vi "Write Voltage Setting.vi"(0 "VISA resource name":refnum<visa-resource-name>, 1 "Enable Voltage Inversion (T: Enabled)":bool=TRUE, 7 "Voltage Setting (100.00)":dbl=100.0 format="%.2f", 11 "error in (no error)":errorcluster) -> (4 "VISA resource name out":refnum<visa-resource-name>, 15 "error out":errorcluster)   [LabVIEW 2011, in "Stanford Research PS300 Series.lvlib"]
doc: "This VI sets the output value and causes the instrument to output voltage."
uses:
  <instrlib>/Stanford Research PS300 Series/Stanford Research PS300 Series.lvlib
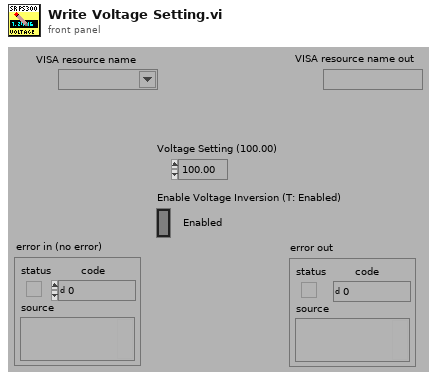
[diagram p1: front panel]
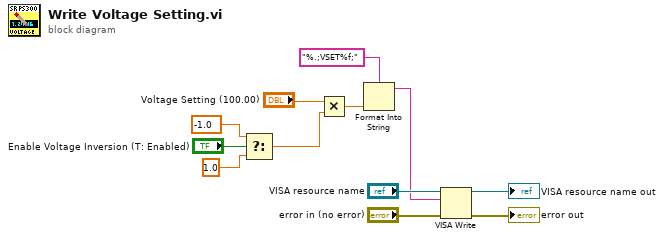
[diagram p0: block diagram]
diagram:
  n1 = Select(t=-1.0 ("y"), s="Enable Voltage Inversion (T: Enabled)", f=1.0) -> (s? t:f=w1:dbl)
  n2 = Multiply(x="Voltage Setting (100.00)", y=w1) -> (x*y=w5:dbl)
  n3 = Format Into String(format string="%.;VSET%f;", w5) -> (resulting string=w8:string)  [unwired: 2 in, 1 out]
  n4 = VISA Write(VISA resource name="VISA resource name", write buffer=w8, error in (no error)="error in (no error)") -> (VISA resource name out=→"VISA resource name out":refnum<visa-resource-name>, error out=→"error out":errorcluster)  [unwired: 1 out]
